vi "Set Error Source.vi"(8 "class name (\"\")":string, 9 "library name (\"\")":string, 10 "vi name":string, 11 "error in":errorcluster) -> (1 "initial offset":i32, 3 "error out":errorcluster)   [LabVIEW 2020, in "Static Errors.lvlib"]
doc: "Sets the source VI, class, and library of <b>error</b>.\n\n<b>Note:</b> This VI should be used before other edits to the error source string are made since it overwrites the existing string starting at byte offset 0."
uses:
  Static Errors.lvlib
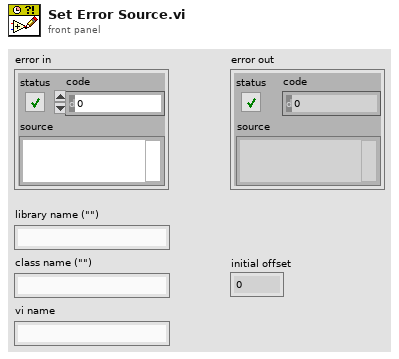
[diagram p1: front panel]
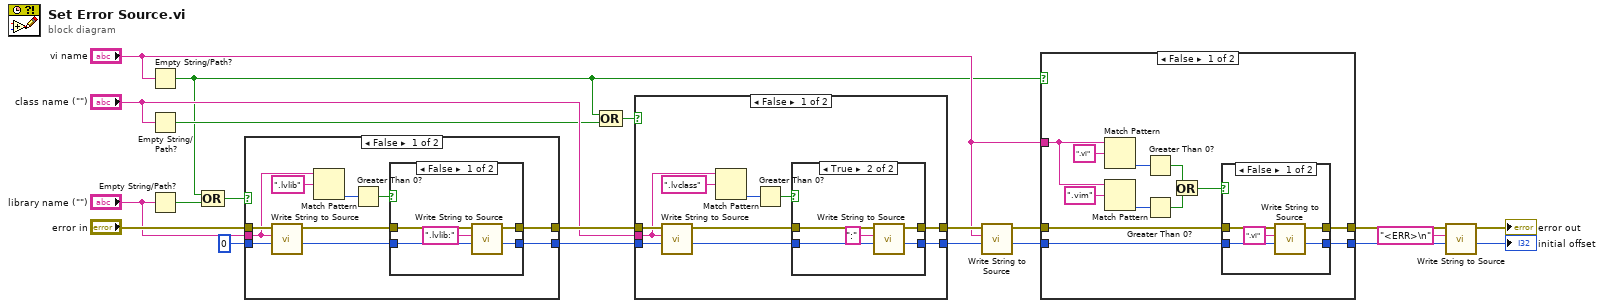
[diagram p0: block diagram]
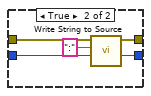
[diagram p2: hidden frame]
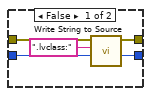
[diagram p4: hidden frame]
diagram:
  n1 = Empty String/Path?(string/path="vi name") -> (empty?=w1:bool)
  n2 = Empty String/Path?(string/path="class name (\"\")") -> (empty?=w2:bool)
  n3 = Empty String/Path?(string/path="library name (\"\")") -> (empty?=w12:bool)
  n4 = Compound Arithmetic op=OR(w1, w12) -> (w11:bool)
  n5 = case shown="False" w11 {
    tunnel: "error in" -> [w31 w43]
    tunnel: 0 ("offset") -> [w30 w42]
    tunnel: [w24 w43] -> w9
    tunnel: [w23 w42] -> w8
    tunnel: "library name (\"\")" -> [w22 _]
    frame False {
      n6 = call "Write String to Source.vi"("offset"=w30, "string"=w22, "error in"=w31) -> ("new offset"=w25:i32, "error out"=w26:errorcluster)  [unwired: 7 in]
      n7 = Match Pattern(string=w22, regular expression=".lvlib") -> (offset past match=w29:i32)  [unwired: 1 in, 3 out]
      n8 = Greater Than 0?(x=w29) -> (x > 0?=w27:bool)
      n9 = case shown="False" w27 {
        tunnel: [w36 w41] -> w24
        tunnel: [w35 w40] -> w23
        tunnel: w26 -> [w33 w38]
        tunnel: w25 -> [w32 w37]
        frame False {
          n10 = call "Write String to Source.vi"("offset"=w32, "string"=".lvlib:", "error in"=w33) -> ("new offset"=w35:i32, "error out"=w36:errorcluster)  [unwired: 7 in]
        }
        frame True {
          n11 = call "Write String to Source.vi"("offset"=w37, "string"=":", "error in"=w38) -> ("new offset"=w40:i32, "error out"=w41:errorcluster)  [unwired: 7 in]
        }
      }
    }
    frame True {
    }
  }
  n12 = Compound Arithmetic op=OR(w1, w2) -> (w10:bool)
  n13 = case shown="False" w10 {
    tunnel: w9 -> [w51 w65]
    tunnel: w8 -> [w50 w64]
    tunnel: [w53 w65] -> w18
    tunnel: [w52 w64] -> w17
    tunnel: "class name (\"\")" -> [w45 _]
    frame False {
      n14 = call "Write String to Source.vi"("offset"=w50, "string"=w45, "error in"=w51) -> ("new offset"=w48:i32, "error out"=w49:errorcluster)  [unwired: 7 in]
      n15 = Match Pattern(string=w45, regular expression=".lvclass") -> (offset past match=w47:i32)  [unwired: 1 in, 3 out]
      n16 = Greater Than 0?(x=w47) -> (x > 0?=w44:bool)
      n17 = case shown="True" w44 {
        tunnel: [w58 w63] -> w53
        tunnel: [w57 w62] -> w52
        tunnel: w49 -> [w55 w60]
        tunnel: w48 -> [w54 w59]
        frame False {
          n18 = call "Write String to Source.vi"("offset"=w54, "string"=".lvclass:", "error in"=w55) -> ("new offset"=w57:i32, "error out"=w58:errorcluster)  [unwired: 7 in]
        }
        frame True {
          n19 = call "Write String to Source.vi"("offset"=w59, "string"=":", "error in"=w60) -> ("new offset"=w62:i32, "error out"=w63:errorcluster)  [unwired: 7 in]
        }
      }
    }
    frame True {
    }
  }
  n20 = call "Write String to Source.vi"("offset"=w17, "string"="vi name", "error in"=w18) -> ("new offset"=w15:i32, "error out"=w16:errorcluster)  [unwired: 7 in]
  n21 = case shown="False" w1 {
    tunnel: w16 -> [w77 w86]
    tunnel: w15 -> [w76 w85]
    tunnel: [w75 w86] -> w14
    tunnel: [w74 w85] -> w13
    tunnel: "vi name" -> [w71 _]
    frame False {
      n22 = Match Pattern(string=w71, regular expression=".vi") -> (offset past match=w70:i32)  [unwired: 1 in, 3 out]
      n23 = Match Pattern(string=w71, regular expression=".vim") -> (offset past match=w69:i32)  [unwired: 1 in, 3 out]
      n24 = Greater Than 0?(x=w70) -> (x > 0?=w67:bool)
      n25 = Greater Than 0?(x=w69) -> (x > 0?=w68:bool)
      n26 = Or(x=w67, y=w68) -> (x .or. y?=w66:bool)
      n27 = case shown="False" w66 {
        tunnel: w77 -> [w82 w84]
        tunnel: w76 -> [w81 w83]
        tunnel: [w80 w84] -> w75
        tunnel: [w79 w83] -> w74
        frame False {
          n28 = call "Write String to Source.vi"("offset"=w81, "string"=".vi", "error in"=w82) -> ("new offset"=w79:i32, "error out"=w80:errorcluster)  [unwired: 7 in]
        }
        frame True {
        }
      }
    }
    frame True {
    }
  }
  n29 = call "Write String to Source.vi"("offset"=w13, "string"="<ERR>\n", "error in"=w14) -> ("new offset"=→"initial offset":i32, "error out"=→"error out":errorcluster)  [unwired: 7 in]
